vi "Add Text Token.vi"(8 "Error In":errorcluster, 11 "Parser In":refnum<class "Parser.lvclass">) -> (0 "Error Out":errorcluster, 3 "Parser Out":refnum<class "Parser.lvclass">)   [LabVIEW 2017, in "Mustache.lvlib" / "Parser.lvclass"]
uses:
  Parser.lvclass
  Parser.lvclass/Parser.ctl
  Tokens/Public/Text/Text.lvclass
  D:/Users/cfield/Code/Field R&D Services/Mustache/feature-lv-original-parser/src/Mustache/Public/Tokens/Public/Abstract/Abstract.lvclass
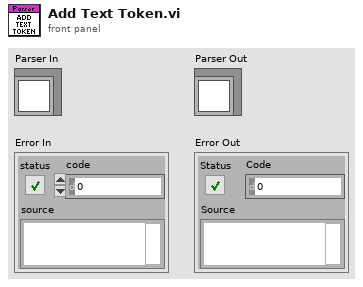
[diagram p1: front panel]
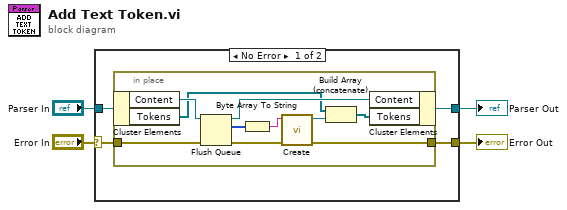
[diagram p0: block diagram]
diagram:
  n1 = case shown="No Error" "Error In" {
    selector: "Error In" -> [w5 w19]
    tunnel: [w8 w19] -> w4
    tunnel: [w7 w20] -> w3
    tunnel: "Parser In" -> [w6 w20]
    frame No Error {
      n2 = in-place {
        in-place-border: [w13] -> w8
        in-place-border: w5 -> [w9]
        n3 = in-place-cluster #1(w6) -> ("Content"=w18:refnum<queue>, "Tokens"=w12:refnum<class "Abstract.lvclass">[])
        n4 = Flush Queue(queue=w18, error in (no error)=w9) -> (queue out=w17:refnum<queue>, remaining elements=w16:u8[], error out=w14:errorcluster)
        n5 = Byte Array To String(unsigned byte array=w16) -> (string=w15:string)
        n6 = call "Create.vi"("Error In"=w14, "Content"=w15) -> ("Error Out"=w13:errorcluster, "Text"=w11:refnum<class "Text.lvclass">)  [unwired: 8 in]
        n7 = Build Array (concatenate)(w12, w11) -> (w10:refnum<class "Abstract.lvclass">[])
        n8 = in-place-cluster #1("Content"=w17, "Tokens"=w10) -> (w7:refnum<class "Parser.lvclass">)
      }
    }
    frame Error {
    }
  }
  "Error Out" <- w4
  "Parser Out" <- w3
